vi "DevRef Data Base fg.vi"(0 "Menu":T12, 1 "Shooter Solenoid DevRef":T8={"DevStatus"={"status"=FALSE, "code"=0, "source"=""}, "Solenoid Module"=enum."Solenoid Module 1", "Forward Solenoid Channel"=enum."Invalid", "Reverse Solenoid Channel"=enum."Invalid"}, 2 "Latch Solenoid DevRef":T8={"DevStatus"={"status"=FALSE, "code"=0, "source"=""}, "Solenoid Module"=enum."Solenoid Module 1", "Forward Solenoid Channel"=enum."Invalid", "Reverse Solenoid Channel"=enum."Invalid"}, 3 "Right Up DevRef":T5={"DevStatus"={"status"=FALSE, "code"=0, "source"=""}, "DIO Channel"=enum."Invalid", "Digital Module"=enum."Digital Module 1"}, 4 "Right Down DevRef":T5={"DevStatus"={"status"=FALSE, "code"=0, "source"=""}, "DIO Channel"=enum."Invalid", "Digital Module"=enum."Digital Module 1"}, 5 "Hold Sensor DevRef":T5={"DevStatus"={"status"=FALSE, "code"=0, "source"=""}, "DIO Channel"=enum."Invalid", "Digital Module"=enum."Digital Module 1"}, 6 "Arm Encoder DevRef":T1={"DevStatus"={"status"=FALSE, "code"=0, "source"=""}, "EncoderIndex"=enum."Invalid", "CounterIndex"=enum."Invalid", "DistancePerCount"=1.0, "Decoding Type"=enum."4x"}, 10 "DevRef to Get":T11) -> (20 "Selected Solenoid":T8={"DevStatus"={"status"=FALSE, "code"=0, "source"=""}, "Solenoid Module"=enum."Solenoid Module 1", "Forward Solenoid Channel"=enum."Invalid", "Reverse Solenoid Channel"=enum."Invalid"}, 21 "Selected Sensor":T5, 22 "Selected Encoder":T1={"DevStatus"={"status"=FALSE, "code"=0, "source"=""}, "EncoderIndex"=enum."Invalid", "CounterIndex"=enum."Invalid", "DistancePerCount"=1.0, "Decoding Type"=enum."4x"})   [LabVIEW 2013]
uses:
  <vilib>/Rock Robotics/WPI/Solenoid/WPI_SolenoidDevRef.ctl
  <vilib>/Rock Robotics/SystemInterfaces/Typedef/FPGA_TypedefSolenoidModule.ctl
  <vilib>/Rock Robotics/WPI/Solenoid/WPI_SolenoidChannel.ctl
  <vilib>/Rock Robotics/WPI/DigitalInput/WPI_DigitalInputDevRef.ctl
  <vilib>/Rock Robotics/SystemInterfaces/DIO/FPGA_DIOChannel.ctl
  <vilib>/Rock Robotics/SystemInterfaces/Typedef/FPGA_TypedefDigitalModule.ctl
  typedefs/fg_typedef.ctl
  UberCode Suffield Philification/typedefs/DevRef Type.ctl
  <vilib>/Rock Robotics/WPI/Encoder/WPI_EncoderDevRef.ctl
  <vilib>/Rock Robotics/SystemInterfaces/Encoder/FPGA_EncoderIdx.ctl
  <vilib>/Rock Robotics/SystemInterfaces/Counter/FPGA_CounterCtrSystemIndex.ctl
  <vilib>/Rock Robotics/WPI/Encoder/WPI_EncoderType.ctl
panel:
  # "A Functional Global that stores refnums for \ncommonly used devices \nso as to not need to get them repeatedly"
  # "it is only set once"
  # "Option to Select Also..."
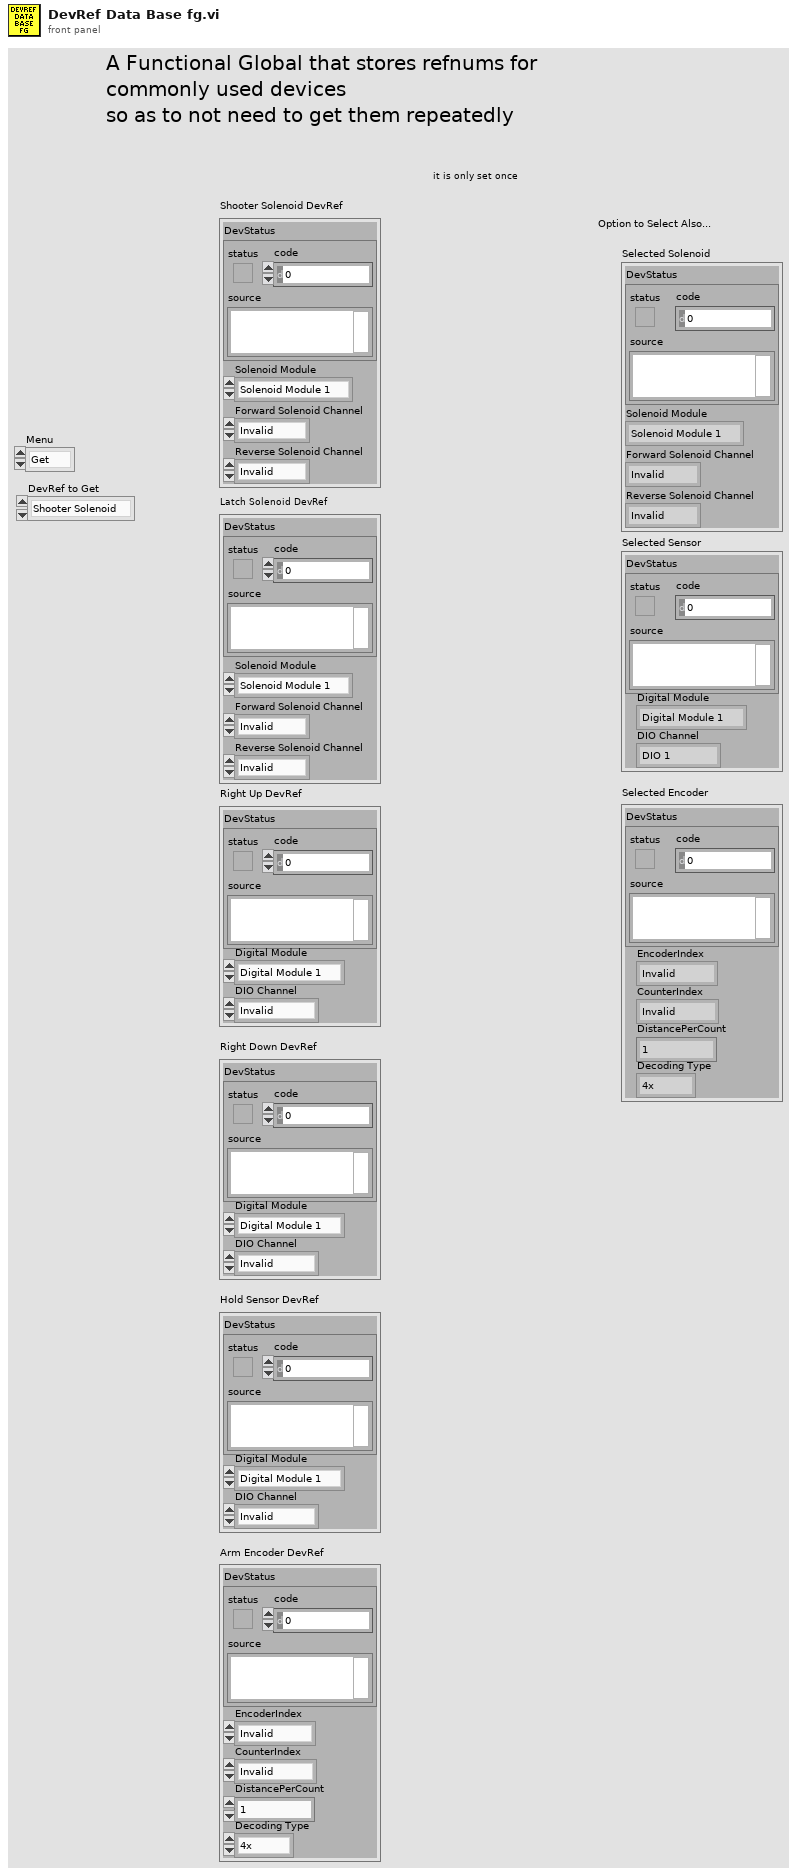
[diagram p1: front panel]
types:
  T1 = typedef "WPI_EncoderDevRef.ctl" = cluster{"DevStatus":errorcluster, "EncoderIndex":T2, "CounterIndex":T3, "DistancePerCount":dbl, "Decoding Type":T4}
  T2 = typedef "FPGA_EncoderIdx.ctl" = enum8{"Enc 0", "Enc 1", "Enc 2", "Enc 3", "Invalid"}
  T3 = typedef "FPGA_CounterCtrSystemIndex.ctl" = enum8{"Ctr 0", "Ctr 1", "Ctr 2", "Ctr 3", "Ctr 4", "Ctr 5", "Ctr 6", "Ctr 7", "Invalid"}
  T4 = typedef "WPI_EncoderType.ctl" = enum16{"1x", "2x", "4x"}
  T5 = typedef "WPI_DigitalInputDevRef.ctl" = cluster{"DevStatus":errorcluster, "DIO Channel":T6, "Digital Module":T7}
  T6 = typedef "FPGA_DIOChannel.ctl" = enum8{"DIO 1", "DIO 2", "DIO 3", "DIO 4", "DIO 5", "DIO 6", "DIO 7", "DIO 8", "DIO 9", "DIO 10", "DIO 11", "DIO 12", "DIO 13", "DIO 14", "Invalid"}
  T7 = typedef "FPGA_TypedefDigitalModule.ctl" = enum16{"Digital Module 1", "Digital Module 2"}
  T8 = typedef "WPI_SolenoidDevRef.ctl" = cluster{"DevStatus":errorcluster, "Solenoid Module":T9, "Forward Solenoid Channel":T10, "Reverse Solenoid Channel":T10}
  T9 = typedef "FPGA_TypedefSolenoidModule.ctl" = enum16{"Solenoid Module 1", "Solenoid Module 2"}
  T10 = typedef "WPI_SolenoidChannel.ctl" = enum8{"Solenoid 1", "Solenoid 2", "Solenoid 3", "Solenoid 4", "Solenoid 5", "Solenoid 6", "Solenoid 7", "Solenoid 8", "Invalid"}
  T11 = typedef "DevRef Type.ctl" = enum16{"Shooter Solenoid", "Latch Solenoid", "Right Up Sensor", "Right Down Sensor", "Hold Sensor", "Arm Encoder"}
  T12 = typedef "fg_typedef.ctl" = enum16{"Get", "Set"}
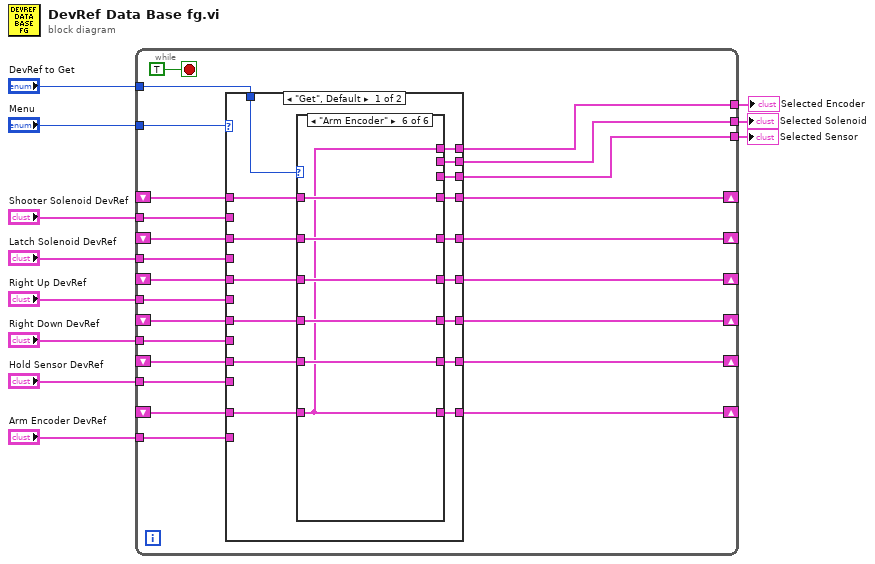
[diagram p0: block diagram]
diagram:
  n1 = while {
    shift-right: [w29] -> _
    shift-left: _ -> [w34]
    shift-right: [w28] -> _
    shift-left: _ -> [w33]
    shift-right: [w27] -> _
    shift-left: _ -> [w31]
    shift-right: [w26] -> _
    shift-left: _ -> [w30]
    tunnel: "Menu" -> [w32]
    tunnel: "Shooter Solenoid DevRef" -> [w25]
    tunnel: "Latch Solenoid DevRef" -> [w24]
    tunnel: "Right Up DevRef" -> [w23]
    tunnel: "Right Down DevRef" -> [w22]
    shift-right: [w19] -> _
    shift-left: _ -> [w20]
    tunnel: "Hold Sensor DevRef" -> [w21]
    tunnel: "DevRef to Get" -> [w18]
    tunnel: [w17] -> w4
    tunnel: [w16] -> w3
    tunnel: "Arm Encoder DevRef" -> [w15]
    shift-right: [w13] -> _
    shift-left: _ -> [w14]
    tunnel: [w12] -> w1
    stop <- TRUE stop-if-true
    n2 = case shown="\"Get\", Default" w32 {
      tunnel: w34 -> [w50 _]
      tunnel: w33 -> [w49 _]
      tunnel: w31 -> [w48 _]
      tunnel: w30 -> [w47 _]
      tunnel: [w39 w93] -> w29
      tunnel: [w40 w92] -> w28
      tunnel: [w41 w91] -> w27
      tunnel: [w42 w90] -> w26
      tunnel: w25 -> [_ w93]
      tunnel: w24 -> [_ w92]
      tunnel: w23 -> [_ w91]
      tunnel: w22 -> [_ w90]
      tunnel: w21 -> [_ w89]
      tunnel: w20 -> [w46 _]
      tunnel: [w43 w89] -> w19
      tunnel: w18 -> [w51 _]
      tunnel: [w45 _] -> w17
      tunnel: [w44 _] -> w16
      tunnel: w15 -> [_ w88]
      tunnel: w14 -> [w38 _]
      tunnel: [w37 w88] -> w13
      tunnel: [w36 _] -> w12
      frame "Get", Default {
        n3 = case shown="\"Arm Encoder\"" w51 {
          tunnel: w50 -> [w53 w63 w69 w75 w81 w87]
          tunnel: w49 -> [w54 w62 w68 w74 w80 w86]
          tunnel: w48 -> [w55 w61 w67 w73 w79 w85]
          tunnel: w47 -> [w56 w60 w66 w72 w78 w84]
          tunnel: w46 -> [w57 w59 w65 w71 w77 w83]
          tunnel: [w53 w62 _ _ _ _] -> w45
          tunnel: [_ _ w67 w72 w77 _] -> w44
          tunnel: [w57 w59 w65 w71 w77 w83] -> w43
          tunnel: [w56 w60 w66 w72 w78 w84] -> w42
          tunnel: [w55 w61 w67 w73 w79 w85] -> w41
          tunnel: [w54 w62 w68 w74 w80 w86] -> w40
          tunnel: [w53 w63 w69 w75 w81 w87] -> w39
          tunnel: w38 -> [w52 w58 w64 w70 w76 w82]
          tunnel: [w52 w58 w64 w70 w76 w82] -> w37
          tunnel: [_ _ _ _ _ w82] -> w36
          frame "Shooter Solenoid", Default {
          }
          frame "Latch Solenoid" {
          }
          frame "Right Up Sensor" {
          }
          frame "Right Down Sensor" {
          }
          frame "Hold Sensor" {
          }
          frame "Arm Encoder" {
          }
        }
      }
      frame "Set" {
      }
    }
  }
  "Selected Solenoid" <- w4
  "Selected Sensor" <- w3
  "Selected Encoder" <- w1
